vi "channel list helper.vi"(8 "Value":string, 9 "Coords":T1, 10 "Table In":refnum<vi>, 11 "Function":T2) -> (0 "error out":errorcluster, 1 "Value":string, 2 "Column":i32, 3 "Row":i32)   [LabVIEW 2013, in "fixed channel tag bus module editor node.lvclass"]
uses:
  fixed channel tag bus module editor node.lvclass
  channel list helper functions.ctl
  <vilib>/Utility/miscctls.llb/LVPoint32TypeDef.ctl
  <vilib>/Utility/miscctls.llb/LVRowAndColumnTypeDef.ctl
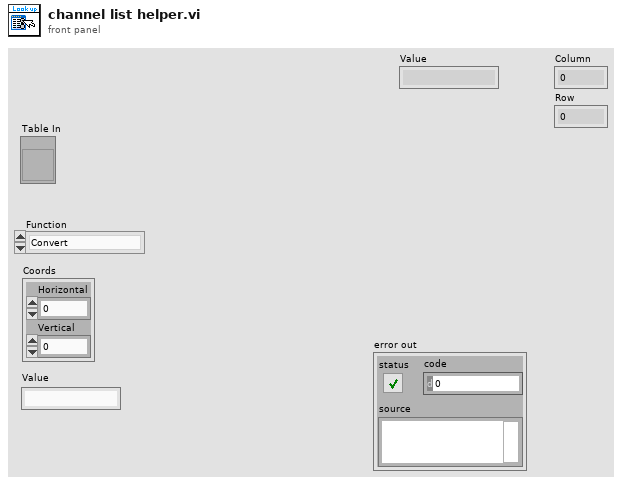
[diagram p1: front panel]
types:
  T1 = typedef "LVPoint32TypeDef.ctl" = cluster{"Horizontal":i32, "Vertical":i32}
  T2 = typedef "fixed channel tag bus module editor node.lvclass/channel list helper functions.ctl" = enum16{"Convert", "Get Value", "Update Value", "Analyze Table"}
  T3 = typedef "LVRowAndColumnTypeDef.ctl" = cluster{"Row":i32, "Column":i32}
  T4 = typedef "LVRowAndColumnUnsignedTypeDef.ctl" = cluster{"Row":u32, "Column":u32}
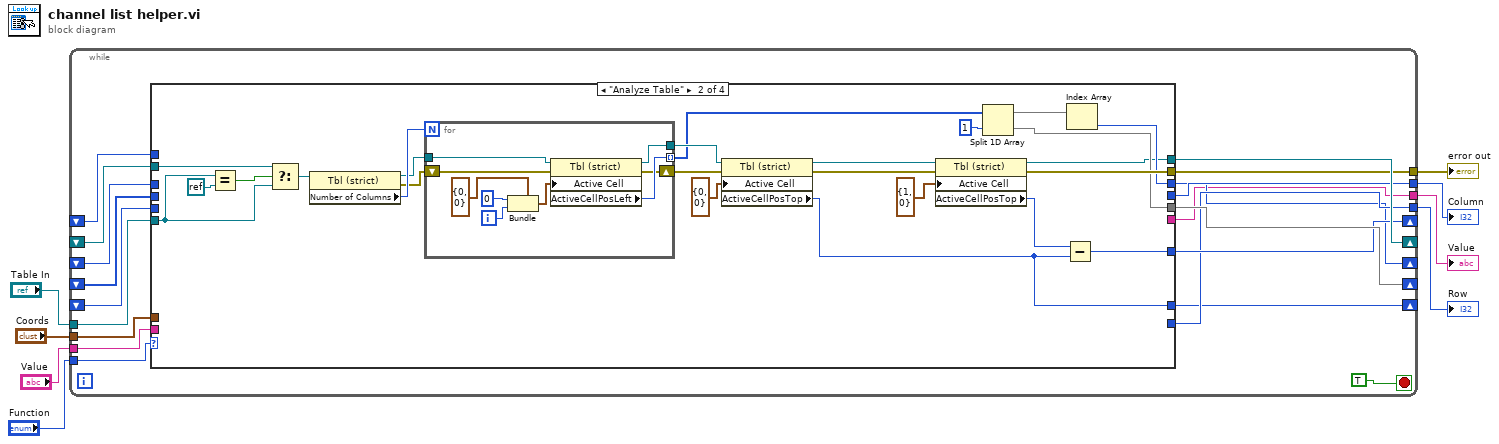
[diagram p0: block diagram]
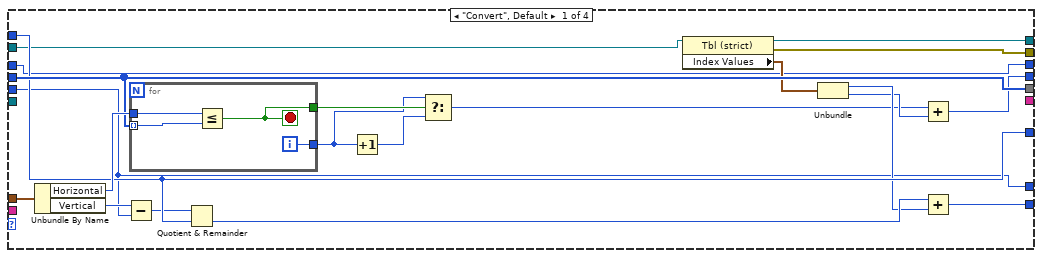
[diagram p2: hidden frame]
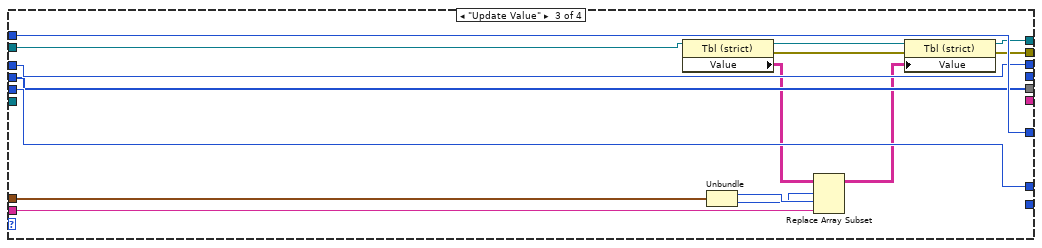
[diagram p3: hidden frame]
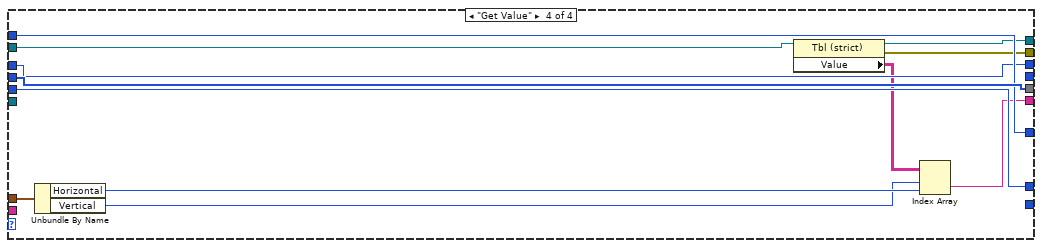
[diagram p4: hidden frame]
diagram:
  n1 = while {
    tunnel: "Function" -> [w27]
    shift-right: [w25] -> _
    shift-left: _ -> [w26]
    shift-right: [w24] -> _
    shift-left: _ -> [w19]
    shift-right: [w23] -> _
    shift-left: _ -> [w17]
    tunnel: [w22] -> w7
    tunnel: "Coords" -> [w21]
    tunnel: "Table In" -> [w20]
    tunnel: [w18] -> w4
    tunnel: [w16] -> w3
    shift-right: [w14] -> _
    shift-left: _ -> [w13]
    shift-right: [w12] -> _
    shift-left: _ -> [w11]
    tunnel: "Value" -> [w10]
    tunnel: [w9] -> w1
    stop <- TRUE stop-if-true
    n2 = case shown="\"Analyze Table\"" w27 {
      tunnel: w26 -> [w43 w67 w96 w101]
      tunnel: [w28 w53 w87 w103] -> w25
      tunnel: [w45 w54 w97 w112] -> w24
      tunnel: [w44 w65 w99 w111] -> w23
      tunnel: [w29 w61 w86 w102] -> w22
      tunnel: w21 -> [w48 _ w94 w107]
      tunnel: w20 -> [_ w60 _ _]
      tunnel: w19 -> [w45 _ w97 w112]
      tunnel: [w37 _ _ _] -> w18
      tunnel: w17 -> [w44 _ w99 w111]
      tunnel: [w39 _ _ _] -> w16
      tunnel: [w30 w59 w100 w109] -> w14
      tunnel: w13 -> [w30 _ w100 w109]
      tunnel: [w34 w55 w98 w110] -> w12
      tunnel: w11 -> [w34 _ w98 w110]
      tunnel: w10 -> [_ _ w91 _]
      tunnel: [_ _ _ w104] -> w9
      frame "Convert", Default {
        n3 = Unbundle By Name(w48) -> ("Horizontal"=w47:i32, "Vertical"=w46:i32)
        n4 = Subtract(x=w46, y=w30) -> (x-y=w31:i32)
        n5 = for {
          tunnel: w45 -> [w51] mode=indexing
          tunnel: w47 -> [w50]
          tunnel: [w52] -> w33
          tunnel: [w49] -> w36
          i -> [w52]
          stop <- w49 stop-if-true
          n6 = Less Or Equal?(x=w50, y=w51) -> (x <= y?=w49:bool)
        }
        n7 = Quotient & Remainder(x=w31, y=w44) -> (floor(x/y)=w41:i32)  [unwired: 1 out]
        n8 = Increment(x=w33) -> (x+1=w32:i32)
        n9 = Select(t=w33, s=w36, f=w32) -> (s? t:f=w35:i32)
        n10 = property class="Tbl (strict)"(reference=w43) -> (reference out=w28:refnum<vi>, error out=w29:errorcluster, "Index Values"=w42:T4)  [unwired: 1 in]
        n11 = Unbundle(w42) -> ("Row"=w40:u32, "Column"=w38:u32)
        n12 = Add(x=w35, y=w38) -> (x+y=w37:u32)
        n13 = Add(x=w41, y=w40) -> (x+y=w39:u32)
      }
      frame "Analyze Table" {
        n14 = Equal?(x=w60, y=refnum<k0> refnum) -> (x = y?=w68:bool)
        n15 = Select(t=w67, s=w68, f=w60) -> (s? t:f=w66:refnum<vi>)
        n16 = property class="Tbl (strict)"(reference=w66) -> (reference out=w70:refnum<vi>, error out=w64:errorcluster, "Number of Columns"=w76:u32)  [unwired: 1 in]
        n17 = for {
          N: w76 -> [_]
          tunnel: [w81] -> w58 mode=indexing
          tunnel: [w80] -> w75
          tunnel: w70 -> [w79]
          shift-right: [w77] -> w63
          shift-left: w64 -> [w78]
          i -> [w84]
          n18 = Bundle(cluster=T3 {"Row"=0, "Column"=0} ("Active Cell:Active Cell"), "Row"=0, "Column"=w84) -> (w85:T3)
          n19 = property class="Tbl (strict)"(reference=w79, error in=w78, "Active Cell"=w85) -> (reference out=w80:refnum<vi>, error out=w77:errorcluster, "ActiveCellPosLeft"=w81:i32)
        }
        n20 = property class="Tbl (strict)"(reference=w75, error in=w63, "Active Cell"=T3 {"Row"=0, "Column"=0} ("Active Cell:Active Cell")) -> (reference out=w72:refnum<vi>, error out=w62:errorcluster, "ActiveCellPosTop"=w59:i32)
        n21 = property class="Tbl (strict)"(reference=w72, error in=w62, "Active Cell"=T3 {"Row"=1, "Column"=0} ("Active Cell:Active Cell")) -> (reference out=w53:refnum<vi>, error out=w61:errorcluster, "ActiveCellPosTop"=w71:i32)
        n22 = Split 1D Array(array=w58, index=1) -> (first subarray=w56:i32[], second subarray=w54:i32[])
        n23 = Subtract(x=w71, y=w59) -> (x-y=w65:i32)
        n24 = Index Array(array=w56) -> (element=w55:i32)  [unwired: 1 in]
      }
      frame "Update Value" {
        n25 = property class="Tbl (strict)"(reference=w96) -> (reference out=w90:refnum<vi>, error out=w89:errorcluster, "Value"=w95:string[][])  [unwired: 1 in]
        n26 = Unbundle(w94) -> ("Horizontal"=w93:i32, "Vertical"=w92:i32)
        n27 = Replace Array Subset(array=w95, new element=w91, index (row)=w92, index (col)=w93) -> (w88:string[][])
        n28 = property class="Tbl (strict)"(reference=w90, error in=w89, "Value"=w88) -> (reference out=w87:refnum<vi>, error out=w86:errorcluster)
      }
      frame "Get Value" {
        n29 = Unbundle By Name(w107) -> ("Horizontal"=w106:i32, "Vertical"=w105:i32)
        n30 = property class="Tbl (strict)"(reference=w101) -> (reference out=w103:refnum<vi>, error out=w102:errorcluster, "Value"=w108:string[][])  [unwired: 1 in]
        n31 = Index Array(array=w108, index (row)=w105, index (col)=w106) -> (element=w104:string)
      }
    }
  }
  "error out" <- w7
  "Column" <- w4
  "Row" <- w3
  "Value" <- w1
